vi "Write intensity.vi"(8 "error in (no error)":errorcluster, 10 "intensity":dbl, 11 "ElectrometerController in":refnum<class "ElectrometerController.lvclass">) -> (0 "error out":errorcluster, 3 "ElectrometerController out":refnum<class "ElectrometerController.lvclass">)   [LabVIEW 2016, in "ElectrometerController.lvclass"]
uses:
  ElectrometerController.lvclass
  ElectrometerController.lvclass/ElectrometerController.ctl
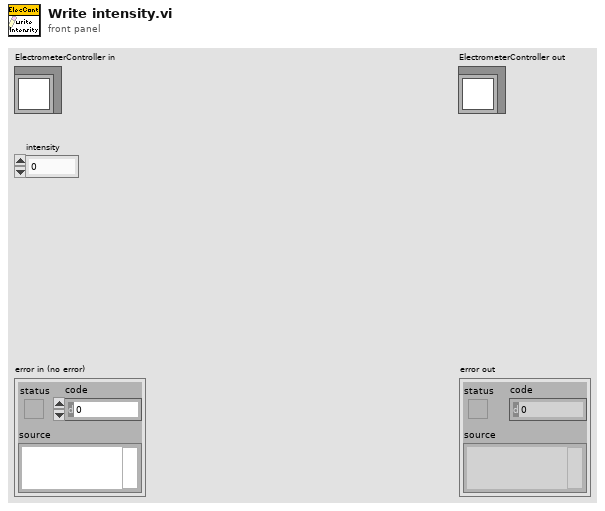
[diagram p1: front panel]
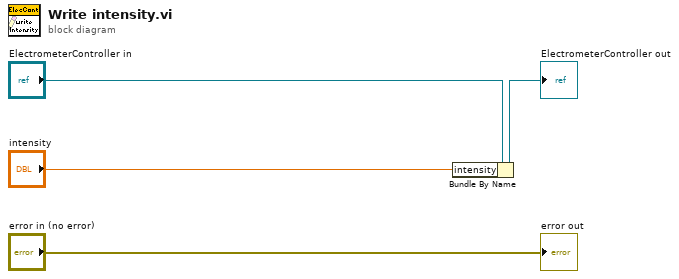
[diagram p0: block diagram]
diagram:
  n1 = Bundle By Name(cluster="ElectrometerController in", "intensity"="intensity") -> (→"ElectrometerController out":refnum<class "ElectrometerController.lvclass">)
  "error out" <- "error in (no error)"
